vi "Batch Convert.vi"(11 "Batch":string) -> (3 "string":string)   [LabVIEW 2015, in "Domino LM.lvlib" / "Domino Laser module Class.lvclass"]
uses:
  Domino Laser module Class.lvclass
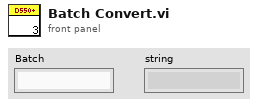
[diagram p1: front panel]
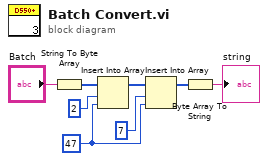
[diagram p0: block diagram]
diagram:
  w6 = u8 47 ("new element/subarray")
  n1 = String To Byte Array(string="Batch") -> (unsigned byte array=w2:u8[])
  n2 = Insert Into Array(array=w2, index=2, new element=w6) -> (w4:u8[])
  n3 = Insert Into Array(array=w4, index=7, new element=w6) -> (w7:u8[])
  n4 = Byte Array To String(unsigned byte array=w7) -> (string=→"string":string)
